vi "Bottle_test.vi"() -> ()   [LabVIEW 2016]
uses:
  <vilib>/Math Plots/2D Math Plots/2D Error Bar/2D Error Bar XCtrl/2D Error Bar.xctl
  <vilib>/Analysis/baseanly.llb/Mean (DBL).vi
  <vilib>/Math Plots/2D Math Plots/2D Error Bar/2D Error Bar Datatype/Public/Plot Helper (Fixed).vi
  <vilib>/Analysis/NI_AALBase.lvlib
  <vilib>/Math Plots/2D Math Plots/2D Error Bar/2D Error Bar Datatype/2D Error Bar Datatype.lvclass
panel:
  in  "Extrapolated":bool=TRUE
  in  "Pulse duration (ms)":dbl format="%#_13g"
  in  "Active bottles":cluster{"String":string, "1":bool}[](array[cluster])
  out "Flow plot":refnum<class "2D Plot Datatype.lvclass">[](xcontrol) caption="2D Error Bar"
  out "Leak plot":refnum<class "2D Plot Datatype.lvclass">[](xcontrol) caption="2D Error Bar"
  out "Status":string
  in  "Repetitions":i32=1
  out "flows":waveform(dbl)[](graph)
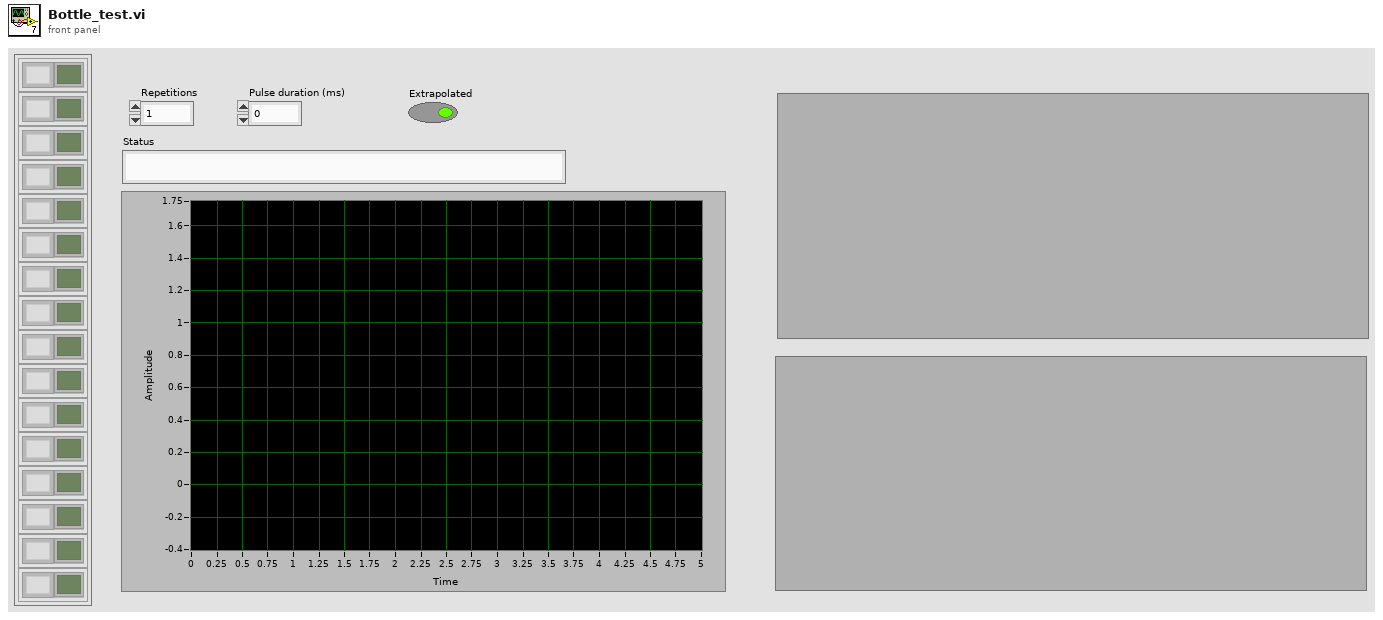
[diagram p1: front panel]
types:
  T1 = enum16{"Leak", "Flow w/o counters", "Flow w counters"}
  T2 = cluster{"Mixture components":cluster{"Name":string, "CID":i32, "Volatility":dbl}[], "Name":string, "VPs":string, "Proportion":cluster{"Numeric":dbl}[], "Selected":bool, "Counter":bool}[][]
  T3 = cluster{"Back valve ON delays":dbl[], "Back valve OFF delays":dbl[], "Step duration (ms)":dbl, "TTL binary step duration (ms)":dbl, "Sampling rate (Hz)":dbl, "Initial delay (ms)":dbl, "Pulse duration (ms)":dbl}
  T4 = typedef "NI_cluster.ctl" = refnum<k21>
  T5 = cluster{"AI task out":refnum<k21>, "DO task out":T4, "AI samples":i32, "Olfactometer parameters":cluster{"Back valve ON delays":dbl[], "Back valve OFF delays":dbl[], "Step duration (ms)":dbl, "TTL binary step duration (ms)":dbl, "Sampling rate (Hz)":dbl, "Initial delay (ms)":dbl, "Pulse duration (ms)":dbl}}
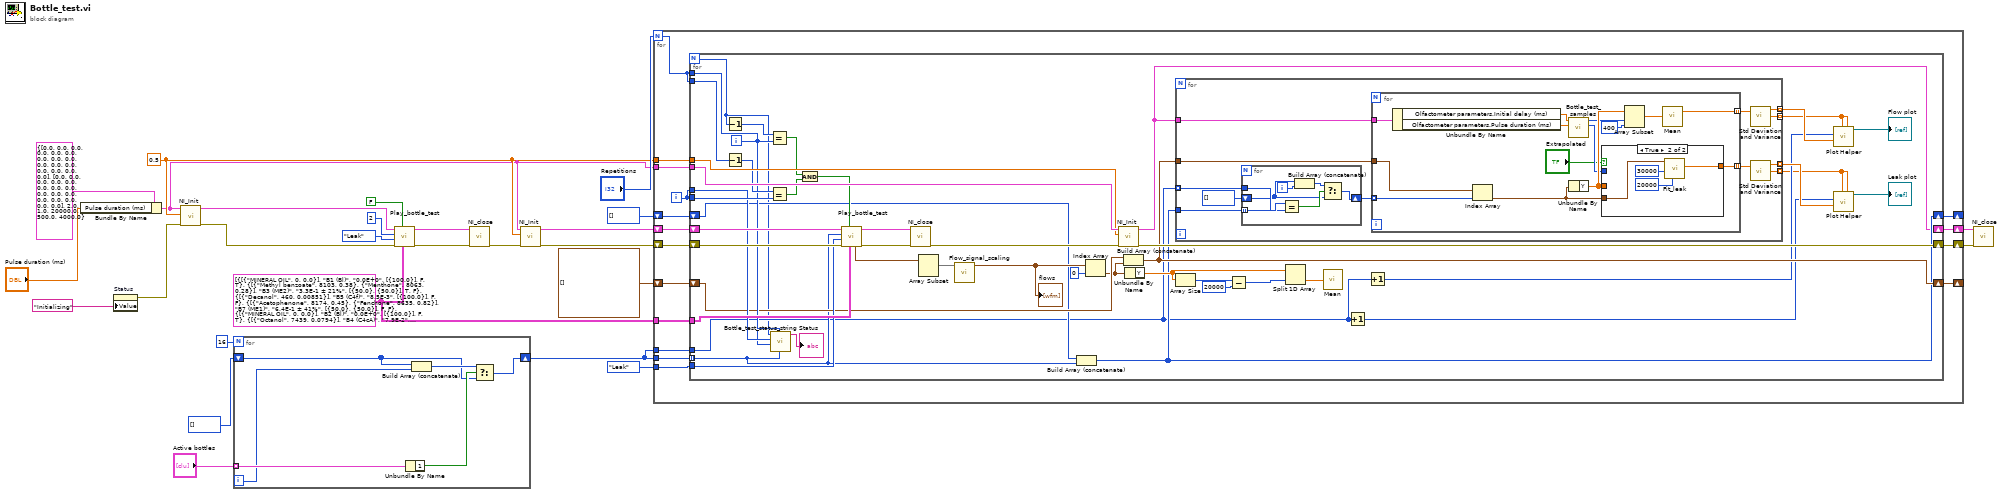
[diagram p0: block diagram]
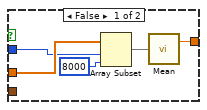
[diagram p2: hidden frame]
diagram:
  w5 = 0.5
  w19 = T2 [[{"Mixture components"=[{"Name"="MINERAL OIL", "CID"=0, "Volatility"=0.0}], "Name"="B1 (Bl)", "VPs"="0.0E+0", "Proportion"=[{"Numeric"=100.0}], "Selected"=FALSE, "Counter"=TRUE}, {"Mixture components"=[{"Name"="Methyl benzoate", "CID"=8103, "Volatility"=0.38}, {"Name"="Menthone", "CID"=8063, "Volatility"=0.28}], "Name"="B3 (ME2)", "VPs"="3.3E-1 ± 21%", "Proportion"=[{"Numeric"=50.0}, {"Numeric"=50.0}], "Selected"=TRUE, "Counter"=FALSE}, {"Mixture components"=[{"Name"="Decanol", "CID"=460, "Volatility"=0.00851}], "Name"="B5 (C4f)", "VPs"="8.5E-3", "Proportion"=[{"Numeric"=100.0}], "Selected"=FALSE, "Counter"=FALSE}, {"Mixture components"=[{"Name"="Acetophenone", "CID"=8174, "Volatility"=0.45}, {"Name"="Fenchone", "CID"=8635, "Volatility"=0.82}], "Name"="B7 (ME1)", "VPs"="6.4E-1 ± 41%", "Proportion"=[{"Numeric"=50.0}, {"Numeric"=50.0}], "Selected"=FALSE, "Counter"=FALSE}], [{"Mixture components"=[{"Name"="MINERAL OIL", "CID"=0, "Volatility"=0.0}], "Name"="B2 (Bl)", "VPs"="0.0E+0", "Proportion"=[{"Numeric"=100.0}], "Selected"=FALSE, "Counter"=TRUE}, {"Mixture components"=[{"Name"="Octanol", "CID"=7439, "Volatility"=0.0794}], "Name"="B4 (C4cA)", "VPs"="7.9E-2", "Proportion"=[{"Numeric"=100.0}], "Selected"=FALSE, "Counter"=FALSE}, {"Mixture components"=[{"Name"="MINERAL OIL", "CID"=0, "Volatility"=0.0}], "Name"="B6 (Bl)", "VPs"="0.0E+0", "Proportion"=[{"Numeric"=100.0}], "Selected"=FALSE, "Counter"=FALSE}, {"Mixture components"=[{"Name"="Heptanoic acid ", "CID"=957, "Volatility"=0.0107}], "Name"="B8 (C3cA)", "VPs"="1.1E-2", "Proportion"=[{"Numeric"=100.0}], "Selected"=FALSE, "Counter"=FALSE}], [{"Mixture components"=[{"Name"="MINERAL OIL", "CID"=0, "Volatility"=0.0}], "Name"="B9 (Bl)", "VPs"="0.0E+0", "Proportion"=[{"Numeric"=100.0}], "Selected"=FALSE, "Counter"=TRUE}, {"Mixture components"=[{"Name"="Geranyl acetate", "CID"=6985, "Volatility"=0.03}, {"Name"="Dimethylacetophenone", "CID"=7144, "Volatility"=0.063}], "Name"="B11 (MW1)", "VPs"="4.6E-2 ± 50%", "Proportion"=[{"Numeric"=50.0}, {"Numeric"=50.0}], "Selected"=FALSE, "Counter"=FALSE}, {"Mixture components"=[{"Name"="Geraniol", "CID"=6405, "Volatility"=0.03}, {"Name"="Phenyl butanone", "CID"=7762, "Volatility"=0.1}], "Name"="B13 (MW2)", "VPs"="6.5E-2 ± 76%", "Proportion"=[{"Numeric"=50.0}, {"Numeric"=50.0}], "Selected"=FALSE, "Counter"=FALSE}, {"Mixture components"=[{"Name"="Methylheptanoic acid", "CID"=1032, "Volatility"=0.018}], "Name"="B15 (C3f)", "VPs"="1.8E-2", "Proportion"=[{"Numeric"=100.0}], "Selected"=FALSE, "Counter"=FALSE}], [{"Mixture components"=[{"Name"="MINERAL OIL", "CID"=0, "Volatility"=0.0}], "Name"="B10 (Bl)", "VPs"="0.0E+0", "Proportion"=[{"Numeric"=100.0}], "Selected"=FALSE, "Counter"=TRUE}, {"Mixture components"=[{"Name"="Valeric acid", "CID"=8025, "Volatility"=0.196}], "Name"="B12 (C3cB)", "VPs"="2.0E-1", "Proportion"=[{"Numeric"=100.0}], "Selected"=FALSE, "Counter"=FALSE}, {"Mixture components"=[{"Name"="Nonanol", "CID"=4133, "Volatility"=0.0227}], "Name"="B14 (C4cB)", "VPs"="2.3E-2", "Proportion"=[{"Numeric"=100.0}], "Selected"=FALSE, "Counter"=FALSE}, {"Mixture components"=[{"Name"="Hydroxacetophenone", "CID"=7462, "Volatility"=0.0856}], "Name"="B16 (Ol)", "VPs"="8.6E-2", "Proportion"=[{"Numeric"=100.0}], "Selected"=FALSE, "Counter"=FALSE}]] ("Odour bottles")
  n1 = Bundle By Name(cluster=T3 {"Back valve ON delays"=[0.0, 0.0, 0.0, 0.0, 0.0, 0.0, 0.0, 0.0, 0.0, 0.0, 0.0, 0.0, 0.0, 0.0, 0.0, 0.0], "Back valve OFF delays"=[0.0, 0.0, 0.0, 0.0, 0.0, 0.0, 0.0, 0.0, 0.0, 0.0, 0.0, 0.0, 0.0, 0.0, 0.0, 0.0], "Step duration (ms)"=2.0, "TTL binary step duration (ms)"=1.0, "Sampling rate (Hz)"=20000.0, "Initial delay (ms)"=500.0, "Pulse duration (ms)"=4000.0} ("Olfactometer parameters"), "Pulse duration (ms)"="Pulse duration (ms)") -> (w3:T3)
  n2 = property on="Status" class="Str"("Value"="Initializing" ("Status")) -> (error out=w10:errorcluster)  [unwired: 2 in, 1 out]
  n3 = call "NI_Init.vi"("error in (no error)"=w10, "Analog input sampling time (s)"=w5, "Olfactometer parameters"=w3) -> ("error out"=w22:errorcluster, "NI cluster out"=w23:T5)  [unwired: 4 in]
  n4 = for {
    N: 16 -> [_]
    tunnel: "Active bottles" -> [w33] mode=indexing
    shift-right: [w31] -> w6
    shift-left: i32[] [] -> [w29]
    i -> [w28]
    n5 = Unbundle By Name(w33) -> ("1"=w32:bool)
    n6 = Build Array (concatenate)(w29, w28) -> (w30:i32[])
    n7 = Select(t=w30, s=w32, f=w29) -> (s? t:f=w31:i32[])
  }
  n8 = call "Play_bottle_test.vi"("Odour bottles"=w19, "Reset counters"=FALSE, "error in (no error)"=w22, "Test type"=T1."Leak", "Tested channel"=2, "NI cluster in"=w23) -> ("error out"=w14:errorcluster, "NI cluster out"=w15:T5)  [unwired: 3 in, 1 out]
  n9 = call "NI_close.vi"("error in (no error)"=w14, "NI cluster in"=w15) -> ("error out"=w13:errorcluster)  [unwired: 9 in]
  n10 = call "NI_Init.vi"("error in (no error)"=w13, "Analog input sampling time (s)"=w5, "Olfactometer parameters"=w3) -> ("error out"=w11:errorcluster, "NI cluster out"=w12:T5)  [unwired: 4 in]
  n11 = for {
    N: "Repetitions" -> [w38]
    tunnel: w19 -> [w47]
    tunnel: T1."Leak" ("Test type") -> [w44]
    tunnel: w6 -> [w43]
    shift-right: [w46] -> w27
    shift-left: w12 -> [w49]
    shift-right: [w45] -> w26
    shift-left: w11 -> [w48]
    tunnel: w3 -> [w42]
    tunnel: w5 -> [w41]
    shift-right: [w40] -> _
    shift-left: waveform(dbl)[] [] -> [w37]
    shift-right: [w36] -> _
    shift-left: i32[] [] -> [w35]
    tunnel: w6 -> [w34]
    i -> [w39]
    n12 = for {
      N -> [w53]
      tunnel: w47 -> [w94]
      tunnel: w44 -> [w93]
      shift-right: [w50] -> w46
      shift-left: w49 -> [w96]
      shift-right: [w85] -> w45
      shift-left: w48 -> [w95]
      tunnel: w43 -> [w66] mode=indexing
      tunnel: w42 -> [w86]
      tunnel: w41 -> [w84]
      tunnel: w39 -> [w76]
      tunnel: w38 -> [w75]
      tunnel: w39 -> [w69]
      tunnel: w38 -> [w54]
      shift-right: [w63] -> w40
      shift-left: w37 -> [w68]
      shift-right: [w62] -> w36
      shift-left: w35 -> [w65]
      tunnel: w34 -> [w60]
      i -> [w70]
      n13 = Decrement(x=w53) -> (x-1=w74:i32)
      n14 = Decrement(x=w75) -> (x-1=w77:i32)
      n15 = Equal?(x=w74, y=w70) -> (x = y?=w73:bool)
      n16 = Equal?(x=w77, y=w76) -> (x = y?=w71:bool)
      n17 = call "Bottle_test_status_string.vi"("curent bottle"=w66, "i of bottles"=w70, "n of repetitions"=w54, "i repetition"=w69, "n of bottles"=w53) -> ("Status"=→"Status":string)  [unwired: 6 in]
      n18 = And(x=w73, y=w71) -> (x .and. y?=w72:bool)
      n19 = call "Play_bottle_test.vi"("Odour bottles"=w94, "Reset counters"=w72, "error in (no error)"=w95, "Test type"=w93, "Tested channel"=w66, "NI cluster in"=w96) -> ("error out"=w82:errorcluster, "NI cluster out"=w83:T5, "AI data"=w79:waveform(dbl)[])  [unwired: 3 in]
      n20 = call "NI_close.vi"("error in (no error)"=w82, "NI cluster in"=w83) -> ("error out"=w81:errorcluster)  [unwired: 9 in]
      n21 = Array Subset(array=w79) -> (w80:waveform(dbl)[])  [unwired: 2 in]
      n22 = call "Flow_signal_scaling.vi"("data"=w80) -> ("Array"=w78:waveform(dbl)[])  [unwired: 10 in]
      "flows" <- w78
      n23 = Build Array (concatenate)(w65, w66) -> (w62:i32[])
      n24 = Index Array(array=w78, index=0) -> (element=w67:waveform(dbl))
      n25 = call "NI_Init.vi"("error in (no error)"=w81, "Analog input sampling time (s)"=w84, "Olfactometer parameters"=w86) -> ("error out"=w85:errorcluster, "NI cluster out"=w50:T5)  [unwired: 4 in]
      n26 = Build Array (concatenate)(w68, w67) -> (w63:waveform(dbl)[])
      n27 = Unbundle By Name(w67) -> ("Y"=w91:dbl[])
      n28 = for {
        tunnel: w63 -> [w108]
        tunnel: w60 -> [w100] mode=indexing
        tunnel: w62 -> [w101]
        tunnel: [w106] -> w61 mode=indexing
        tunnel: [w105] -> w52 mode=indexing
        tunnel: [w103] -> w59 mode=indexing
        tunnel: [w102] -> w58 mode=indexing
        tunnel: w50 -> [w97]
        n29 = for {
          tunnel: w100 -> [w111]
          tunnel: w101 -> [w112] mode=indexing
          shift-right: [w113] -> w98
          shift-left: i32[] [] -> [w109]
          i -> [w115]
          n30 = Equal?(x=w112, y=w111) -> (x = y?=w110:bool)
          n31 = Build Array (concatenate)(w109, w115) -> (w114:i32[])
          n32 = Select(t=w114, s=w110, f=w109) -> (s? t:f=w113:i32[])
        }
        n33 = for {
          tunnel: w98 -> [w129] mode=indexing
          tunnel: w108 -> [w128]
          tunnel: [w127] -> w107 mode=indexing
          tunnel: [w123] -> w104 mode=indexing
          tunnel: w97 -> [w122]
          n34 = Unbundle By Name(w122) -> ("Olfactometer parameters.Initial delay (ms)"=w121:dbl, "Olfactometer parameters.Pulse duration (ms)"=w120:dbl)
          n35 = Index Array(array=w128, index=w129) -> (element=w117:waveform(dbl))
          n36 = call "Bottle_test_samples.vi"("Pulse duration (ms)"=w120, "Initial delay (ms)"=w121) -> ("leak samples start"=w118:i32, "flow samples start"=w119:i32)  [unwired: 8 in]
          n37 = Unbundle By Name(w117) -> ("Y"=w125:dbl[])
          n38 = case shown="True" "Extrapolated" {
            tunnel: [w134 w137] -> w127
            tunnel: w125 -> [w131 _]
            tunnel: w118 -> [w130 _]
            tunnel: w117 -> [_ w138]
            frame False {
              n39 = Array Subset(array=w131, index=w130, length=8000) -> (w132:dbl[])
              n40 = call-poly <vilib>:"Mean.vi"("X"=w132) -> ("mean"=w134:dbl)  [unwired: 1 out]
            }
            frame True {
              n41 = call "Fit_leak.vi"("length"=20000, "start samples/time"=30000, "Waveform"=w138) -> ("Leak (l/min)"=w137:dbl)  [unwired: 7 in, 1 out]
            }
          }
          n42 = Array Subset(array=w125, index=w119, length=400) -> (w124:dbl[])
          n43 = call-poly <vilib>:"Mean.vi"("X"=w124) -> ("mean"=w123:dbl)  [unwired: 1 out]
        }
        n44 = call <vilib>:"Std Deviation and Variance.vi"("X"=w104) -> ("mean"=w103:dbl, "standard deviation"=w102:dbl)  [unwired: 1 in, 1 out]
        n45 = call <vilib>:"Std Deviation and Variance.vi"("X"=w107) -> ("mean"=w106:dbl, "standard deviation"=w105:dbl)  [unwired: 1 in, 1 out]
      }
      n46 = Array Size(array=w91) -> (size(s)=w90:i32)
      n47 = Subtract(x=w90, y=20000) -> (x-y=w88:i32)
      n48 = Split 1D Array(array=w91, index=w88) -> (second subarray=w87:dbl[])  [unwired: 1 out]
      n49 = call-poly <vilib>:"Mean.vi"("X"=w87) -> ()  [unwired: 2 out]
      n50 = Increment(x=w60) -> (x+1=w55:i32[])
      n51 = Increment(x=w60) -> (x+1=w56:i32[])
      n52 = call-poly <vilib>:"Plot Helper.vi"("error b vector"=w58, "error a vector"=w58, "y vector"=w59, "x vector"=w56) -> ("2D Plot Class Obj Array out"=→"Flow plot":refnum<class "2D Plot Datatype.lvclass">[])  [unwired: 2 in, 5 out]
      n53 = call-poly <vilib>:"Plot Helper.vi"("error b vector"=w52, "error a vector"=w52, "y vector"=w61, "x vector"=w55) -> ("2D Plot Class Obj Array out"=→"Leak plot":refnum<class "2D Plot Datatype.lvclass">[])  [unwired: 2 in, 5 out]
    }
  }
  n54 = call "NI_close.vi"("error in (no error)"=w26, "NI cluster in"=w27) -> ()  [unwired: 9 in, 1 out]
